vi "Controls and Indicators.vi"() -> ()   [LabVIEW 2010]
doc: "A sample VI that demonstrates Boolean and string controls and indicators."
panel:
  out "Indicator":string
  in  "Control":string
  out "Indicator":bool
  in  "Control":bool
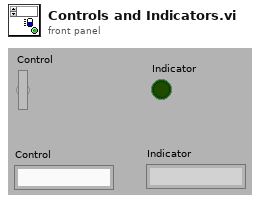
[diagram p1: front panel]
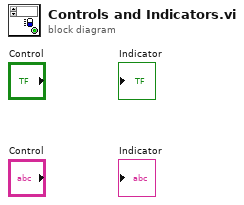
[diagram p0: block diagram]
diagram:
